vi "imu_read.vi"(8 "error in":errorcluster, 11 "VISA resource name":refnum<visa-resource-name>) -> (0 "error out":errorcluster, 1 "checksum error":bool, 2 "data":T1, 3 "VISA resource name out":refnum<visa-resource-name>)   [LabVIEW 2017]
panel:
  in  "data":T1
  out "error":i8
  in  "input mask":T2 {"reserved" format="%x"; "index" format="%x"; "header" format="%x"}
  out "Output String":string
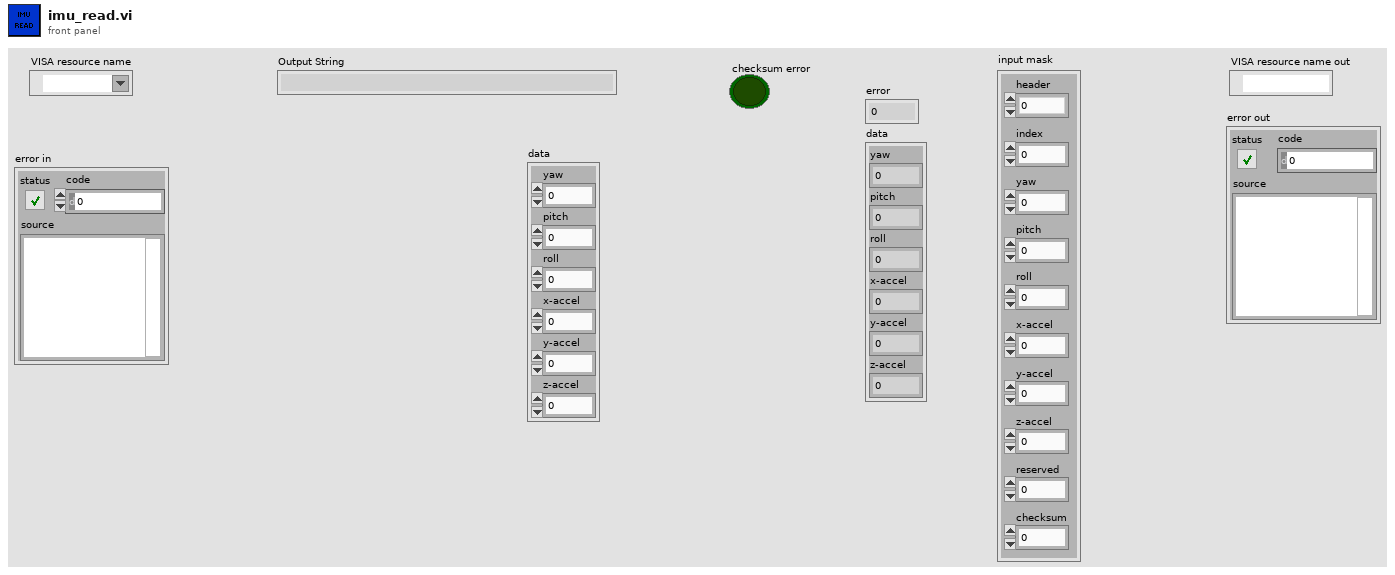
[diagram p1: front panel]
types:
  T1 = cluster{"yaw":dbl, "pitch":dbl, "roll":dbl, "x-accel":dbl, "y-accel":dbl, "z-accel":dbl}
  T2 = cluster{"header":u16, "index":u8, "yaw":i16, "pitch":i16, "roll":i16, "x-accel":i16, "y-accel":i16, "z-accel":i16, "reserved":u16, "checksum":i16}
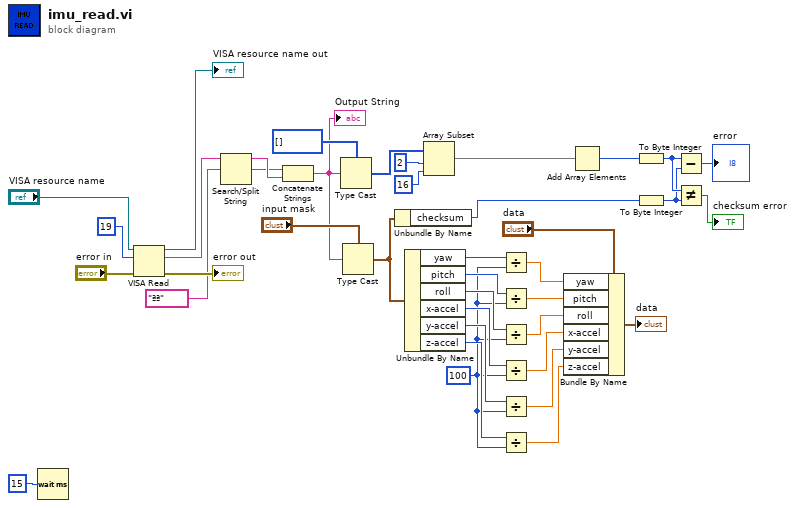
[diagram p0: block diagram]
diagram:
  w2 = i16 100 ("y")
  n1 = Wait (ms)(milliseconds to wait=u32 15) -> ()  [unwired: 1 out]
  n2 = VISA Read(VISA resource name="VISA resource name", byte count=u32 19 ("Character Count"), error in (no error)="error in") -> (VISA resource name out=→"VISA resource name out":refnum<visa-resource-name>, read buffer=w37:string, error out=→"error out":errorcluster)  [unwired: 1 out]
  n3 = Search/Split String(string=w37, search string/char (-)="ªª") -> (substring before match=w36:string, match + rest of string=w35:string)  [unwired: 1 in, 1 out]
  n4 = Concatenate Strings(w35, w36) -> (w1:string)
  "Output String" <- w1
  n5 = Type Cast(type=u8[] [], x=w1) -> (*(type *) &x=w25:u8[])
  n6 = Type Cast(type="input mask", x=w1) -> (*(type *) &x=w17:T2)
  n7 = Unbundle By Name(w17) -> ("checksum"=w24:i16)
  n8 = Unbundle By Name(w17) -> ("yaw"=w15:i16, "pitch"=w14:i16, "roll"=w13:i16, "x-accel"=w12:i16, "y-accel"=w11:i16, "z-accel"=w10:i16)
  n9 = Array Subset(array=w25, index=2, length=16) -> (w26:u8[])
  n10 = Divide(x=w15, y=w2) -> (x/y=w9:dbl)
  n11 = Divide(x=w14, y=w2) -> (x/y=w8:dbl)
  n12 = Divide(x=w13, y=w2) -> (x/y=w7:dbl)
  n13 = Divide(x=w12, y=w2) -> (x/y=w6:dbl)
  n14 = Divide(x=w11, y=w2) -> (x/y=w5:dbl)
  n15 = Divide(x=w10, y=w2) -> (x/y=w4:dbl)
  n16 = Bundle By Name(cluster="data", "yaw"=w9, "pitch"=w8, "roll"=w7, "x-accel"=w6, "y-accel"=w5, "z-accel"=w4) -> (→"data":T1)
  n17 = Add Array Elements(numeric array=w26) -> (sum=w23:u8)
  n18 = To Byte Integer(number=w23) -> (8bit integer=w20:i8)
  n19 = To Byte Integer(number=w24) -> (8bit integer=w19:i8)
  n20 = Subtract(x=w20, y=w19) -> (x-y=→"error":i8)
  n21 = Not Equal?(x=w20, y=w19) -> (x != y?=→"checksum error":bool)
